vi "DDC Stage 01 - 16ch - Does Not Work - for loops.vi"(0 "data in":T1[](array[typedef])=[{"I"=0.0, "Q"=0.0, "overflow"=FALSE}, {"I"=0.0, "Q"=0.0, "overflow"=FALSE}, {"I"=0.0, "Q"=0.0, "overflow"=FALSE}, {"I"=0.0, "Q"=0.0, "overflow"=FALSE}, {"I"=0.0, "Q"=0.0, "overflow"=FALSE}, {"I"=0.0, "Q"=0.0, "overflow"=FALSE}, {"I"=0.0, "Q"=0.0, "overflow"=FALSE}, {"I"=0.0, "Q"=0.0, "overflow"=FALSE}], 1 "acq.reset":bool, 9 "input valid":bool, 11 "Num of channels":u8=16, 12 "ddc.freq.shift":fxp<+/-,48,0>[](array[numeric])=[0.0, 0.0, 0.0, 0.0, 0.0, 0.0, 0.0, 0.0, 0.0, 0.0, 0.0, 0.0, 0.0, 0.0, 0.0, 0.0] format="%.48g", 13 "ddc.phase":fxp<+/-,21,0>[](array[numeric])=[0.0, 0.0, 0.0, 0.0, 0.0, 0.0, 0.0, 0.0, 0.0, 0.0, 0.0, 0.0, 0.0, 0.0, 0.0, 0.0] format="%.21g") -> (3 "CHs overflow":bool[](array[boolean]), 8 "FIFOs Timeout":bool[](array[boolean]))   [LabVIEW 2015, in "DDC_7976R_v1.lvlib"]
uses:
  DDC_7976R_v1.lvlib
  <instrlib>/_niInstr/DSP/v1/Shared/Public/IQ Data.ctl
  <instrlib>/_niInstr/DSP/v1/FPGA/Public/Sub VIs/Frequency Shift/Frequency Shift - 8 spc.vi
  <instrlib>/_niInstr/DSP/v1/Xnodes/Public/Frequency Shift/niInstr DSP v1 Frequency Shift FPGA.xnode
  <instrlib>/_niInstr/DSP/v1/Shared/niInstr DSP v1 Shared.lvlib
  <instrlib>/_niInstr/DSP/v1/FPGA/niInstr DSP v1 FPGA.lvlib
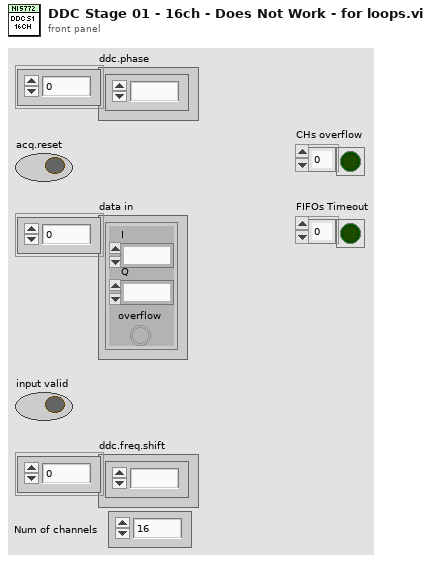
[diagram p1: front panel]
types:
  T1 = typedef "niInstr DSP v1 Shared.lvlib/IQ Data.ctl" = cluster{"I":fxp<+/-,18,1>, "Q":fxp<+/-,18,1>, "overflow":bool}
  T2 = typedef "DDC_7976R_v1.lvlib/16xIQData.ctl" = T1[]
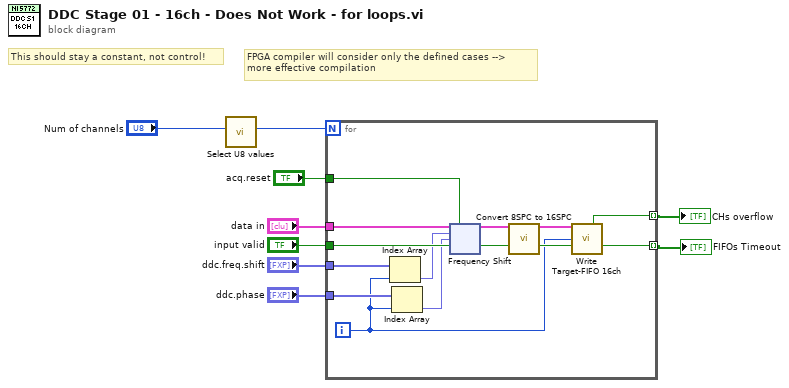
[diagram p0: block diagram]
diagram:
  # "FPGA compiler will consider only the defined cases -->\nmore effective compilation"
  # "This should stay a constant, not control!"
  n1 = call "Select U8 values.vi"("Unput U8"="Num of channels") -> ("output I32"=w5:i32)  [unwired: 10 in]
  n2 = for {
    N: w5 -> [_]
    tunnel: "ddc.phase" -> [w18]
    tunnel: "ddc.freq.shift" -> [w19]
    tunnel: "data in" -> [w20]
    tunnel: "input valid" -> [w21]
    tunnel: [w11] -> w2 mode=indexing
    tunnel: [w12] -> w3 mode=indexing
    tunnel: "acq.reset" -> [w10]
    i -> [w14]
    n3 = Index Array(array=w19, index=w14) -> (element=w17:fxp<+/-,48,0>)
    n4 = Index Array(array=w18, index=w14) -> (element=w16:fxp<+/-,21,0>)
    n5 = xnode "Frequency Shift"("data in"=w20, "reset"=w10, "frequency shift"=w17, "phase"=w16, "input valid"=w21) -> ("data out"=w22:T1[], "output valid"=w23:bool)  [unwired: 1 in, 1 out]
    n6 = call "Convert 8SPC to 16SPC.vi"("8xIQ in"=w22, "input valid"=w23) -> ("16xIQ out"=w13:T2, "output valid"=w15:bool)  [unwired: 12 in]
    n7 = call "Write Target-FIFO 16ch.vi"("16xIQ in"=w13, "Ch select"=w14, "input valid"=w15) -> ("DSP Overflow"=w12:bool, "Timed Out?"=w11:bool)  [unwired: 11 in]
  }
  "FIFOs Timeout" <- w2
  "CHs overflow" <- w3
